vi "Set Progression State.vi"(8 "error in (no error)":errorcluster, 10 "Progression States":T1 items=["No Progression"=0, "Indeterminated"=1, "Normal"=2, "Error"=4, "Paused"=8], 11 "Window Handle":refnum<k24>) -> (0 "error out":errorcluster, 3 "Window Handle out":refnum<k24>)   [LabVIEW 2015, in "Simple Progress Bar.lvlib"]
uses:
  Simple Progress Bar.lvlib
  Window States.ctl
  C:/Program Files (x86)/National Instruments/LabVIEW 2015/vi.lib/TaskbarProgressAPI/Windows7Taskbar.dll
  Program Files (x86)/National Instruments/LabVIEW 2015/vi.lib/TaskbarProgressAPI/Windows7Taskbar.dll
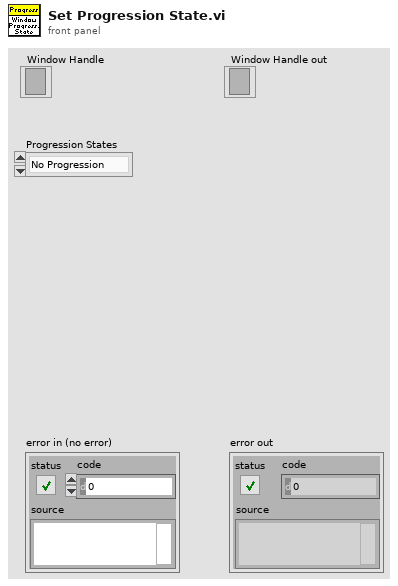
[diagram p1: front panel]
types:
  T1 = typedef "Simple Progress Bar.lvlib/Window States.ctl" = i32
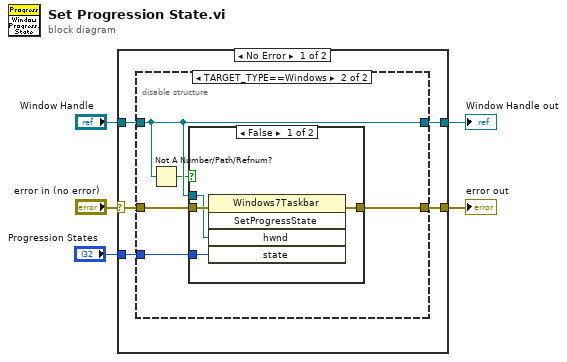
[diagram p0: block diagram]
diagram:
  n1 = case shown="No Error" "error in (no error)" {
    selector: "error in (no error)" -> [w9 w23]
    tunnel: "Window Handle" -> [w10 _]
    tunnel: [w8 w23] -> w4
    tunnel: [w7 _] -> w3
    tunnel: "Progression States" -> [w6 _]
    frame No Error {
      n2 = disable-structure shown="TARGET_TYPE==Windows" {
        disable-tunnel: w10 -> [w11 w14]
        disable-tunnel: w9 -> [w12 w17]
        disable-tunnel: [w12 w15] -> w8
        disable-tunnel: [w11 w14] -> w7
        disable-tunnel: w6 -> [_ w16]
        frame condition #0 {
          # "#ToError"
        }
        frame condition #1 (active) {
          n3 = Not A Number/Path/Refnum?(number/path/refnum=w14) -> (NaN/Path/Refnum?=w13:bool)
          n4 = case shown="False" w13 {
            tunnel: w17 -> [w21 w22]
            tunnel: w16 -> [w20 _]
            tunnel: [w19 w22] -> w15
            tunnel: w14 -> [w18 _]
            frame False {
              n5 = invoke class="Windows7Taskbar" method="SetProgressState"(error in=w21, "hwnd"=w18, "state"=w20) -> (error out=w19:errorcluster)  [unwired: 2 in, 4 out]
            }
            frame True {
            }
          }
        }
      }
    }
    frame Error {
    }
  }
  "error out" <- w4
  "Window Handle out" <- w3
